vi "util_generate_error.vi"(6 "show_call_chain":bool=TRUE, 8 "error in (no error)":errorcluster, 10 "data":variant, 11 "error":T1) -> (0 "error out":errorcluster)   [LabVIEW 2015, in "lv-recipe-machine.lvlib"]
doc: "This VI can be used to generate custom errors and communicate to users when something wrong has happened via an error wire. It is public and can be used to compare errors to clear or ginore."
uses:
  lv-recipe-machine.lvlib
  _controls/error.ctl
  _controls/input_command.ctl
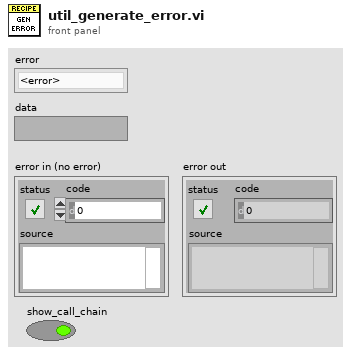
[diagram p1: front panel]
types:
  T1 = typedef "lv-recipe-machine.lvlib/error.ctl" = enum16{"<error>", "bad_command", "command_queue_timeout", "stop_notifier_timeout", "die_command_timeout", "not_in_manual_mode", "not_in_automatic_mode", "not_in_automatic_idle", "not_in_automatic_running", "not_in_automatic_paused", "automatic_step_not_found", "manual_step_not_found", "<null>"}
  T2 = typedef "lv-recipe-machine.lvlib/input_command.ctl" = enum8{"<input_command>", "die", "<null>"}
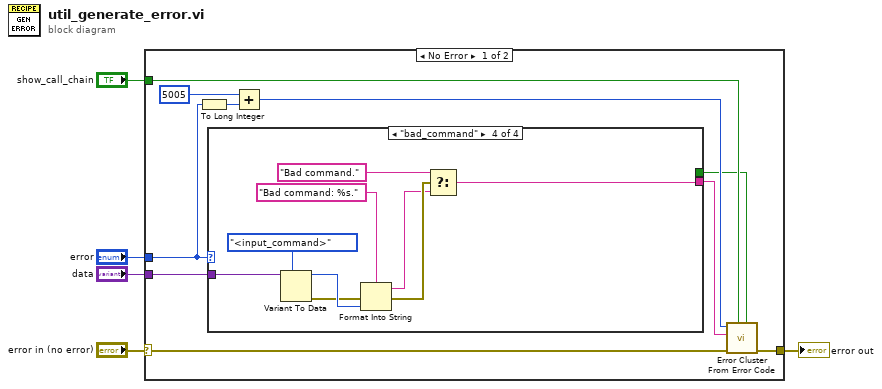
[diagram p0: block diagram]
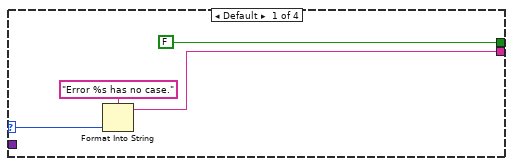
[diagram p2: hidden frame]
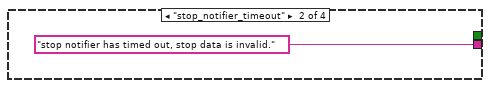
[diagram p3: hidden frame]
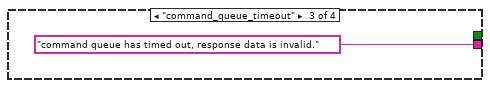
[diagram p4: hidden frame]
diagram:
  n1 = case shown="No Error" "error in (no error)" {
    selector: "error in (no error)" -> [w6 w31]
    tunnel: "data" -> [w15 _]
    tunnel: [w14 w31] -> w3
    tunnel: "error" -> [w12 _]
    tunnel: "show_call_chain" -> [w8 _]
    frame No Error {
      n2 = To Long Integer(number=w12) -> (32bit integer=w11:i32)
      n3 = case shown="\"bad_command\"" w12 {
        selector: w12 -> [w18 _ _ _]
        tunnel: w15 -> [_ _ _ w30]
        tunnel: [w17 "stop notifier has timed out, stop data is invalid." "command queue has timed out, response data is invalid." w25] -> w9
        tunnel: [FALSE _ _ _] -> w7
        frame Default {
          n4 = Format Into String(format string="Error %s has no case.", w18) -> (resulting string=w17:string)  [unwired: 2 in, 1 out]
        }
        frame "stop_notifier_timeout" {
        }
        frame "command_queue_timeout" {
        }
        frame "bad_command" {
          n5 = Variant To Data(type=input_command."<input_command>" ("command"), Variant=w30) -> (data=w28:T2, error out=w27:errorcluster)  [unwired: 1 in]
          n6 = Format Into String(format string="Bad command: %s.", error in=w27, w28) -> (resulting string=w22:string, error out=w26:errorcluster)  [unwired: 1 in]
          n7 = Select(t="Bad command.", s=w26, f=w22) -> (s? t:f=w25:string)
        }
      }
      n8 = Add(x=5005, y=w11) -> (x+y=w10:i32)
      n9 = call <vilib>:"Error Cluster From Error Code.vi"("is warning? (False)"=w7, "show call chain? (False)"=w8, "error in (no error)"=w6, "error message (\"\")"=w9, "error code (0)"=w10) -> ("error out"=w14:errorcluster)  [unwired: 4 in]
    }
    frame Error {
    }
  }
  "error out" <- w3
